vi "期末9-2test.vi"() -> ()   [LabVIEW 2014]
panel:
  out "瞬間尖點座標 2":dbl[][](array[numeric])
  out "尖點座標和 2":dbl[](array[numeric])
  in  "?":bool
  out "number (0 to 1)":dbl
  in  "紀錄中點座標和":bool
  in  "stop":bool
  out "Array":dbl[][](array[numeric])
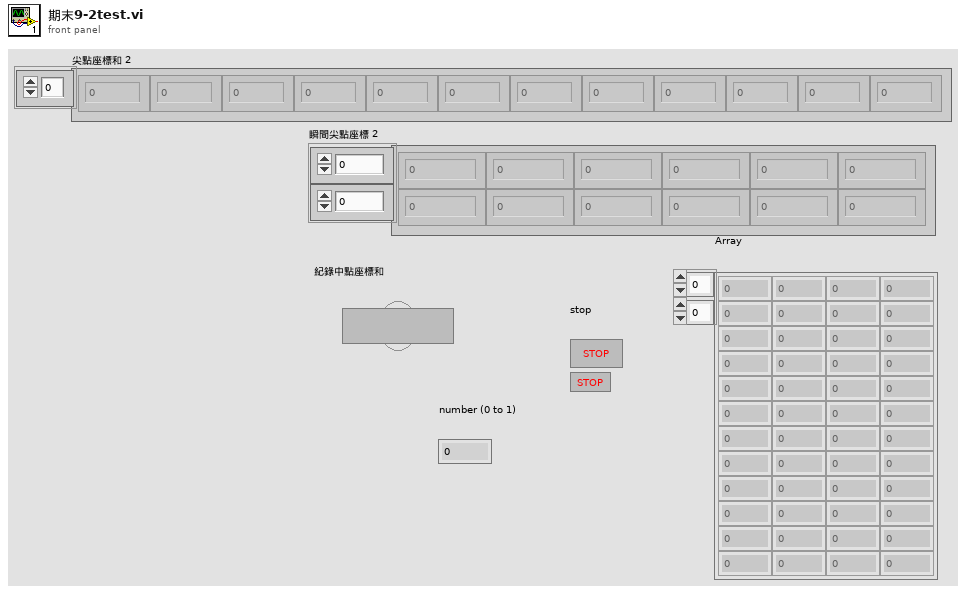
[diagram p1: front panel]
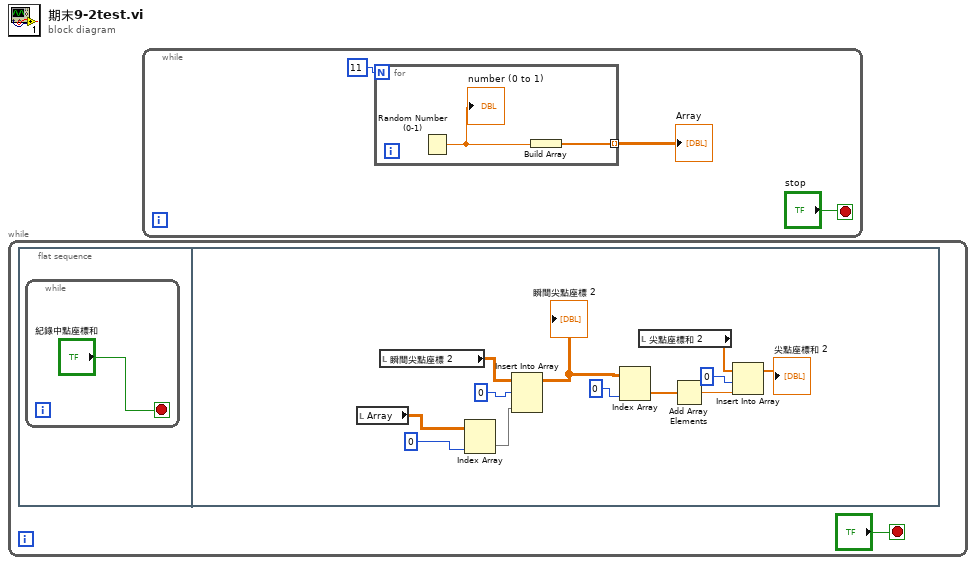
[diagram p0: block diagram]
diagram:
  n1 = while {
    stop <- "?" stop-if-true
    n2 = flat-sequence {
      frame #0 {
        n3 = while {
          stop <- "紀錄中點座標和" stop-if-true
        }
      }
      frame #1 {
        n4 = local read "Array"() -> (w8:dbl[][])
        n5 = local read "瞬間尖點座標 2"() -> (w13:dbl[][])
        n6 = Index Array(array=w8, index (col)=0 ("index (row)")) -> (element=w12:dbl[])  [unwired: 1 in]
        n7 = Insert Into Array "Insert Into Array"(array=w13, index (row)=0 ("index"), new element=w12) -> (w5:dbl[][])  [unwired: 1 in]
        "瞬間尖點座標 2" <- w5
        n8 = Index Array "Index Array"(array=w5, index (col)=0 ("index (row)")) -> (element=w14:dbl[])  [unwired: 1 in]
        n9 = local read "尖點座標和 2"() -> (w9:dbl[])
        n10 = Add Array Elements(numeric array=w14) -> (sum=w4:dbl)
        n11 = Insert Into Array "Insert Into Array"(array=w9, index=0 ("index (row)"), new element=w4) -> (→"尖點座標和 2":dbl[])
      }
    }
  }
  n12 = while {
    stop <- "stop" stop-if-true
    n13 = for {
      N: 11 -> [_]
      tunnel: [w19] -> w16 mode=indexing
      n14 = Random Number (0-1)() -> (number: 0 to 1=w18:dbl)
      "number (0 to 1)" <- w18
      n15 = Build Array(w18) -> (w19:dbl[])
    }
    "Array" <- w16
  }
